vi "performZeroCorrection.vi"(8 "error in (no error)":errorcluster, 9 "Input Range":dbl=10.0 format="%#_10g", 10 "Measurement Function (0: Current)":i32(ring) items=["Current", "Charge", "Voltage", "Resistance"], 11 "Electrometer in":refnum<class "Electrometer.lvclass">) -> (0 "error out":errorcluster, 2 "Set Range":string, 3 "Electrometer out":refnum<class "Electrometer.lvclass">)   [LabVIEW 2016, in "Electrometer.lvclass"]
uses:
  Electrometer.lvclass
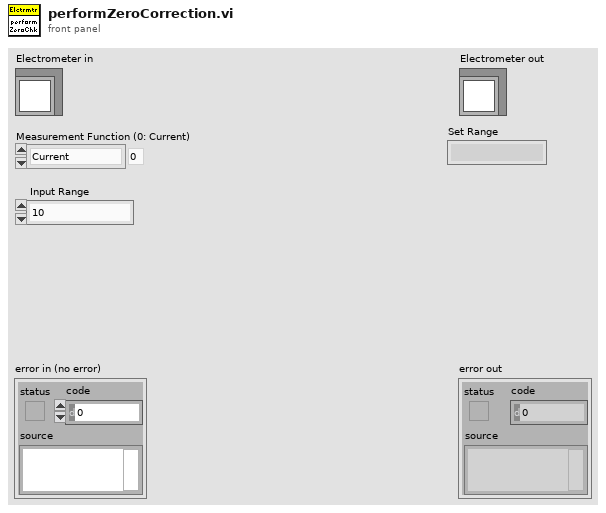
[diagram p1: front panel]
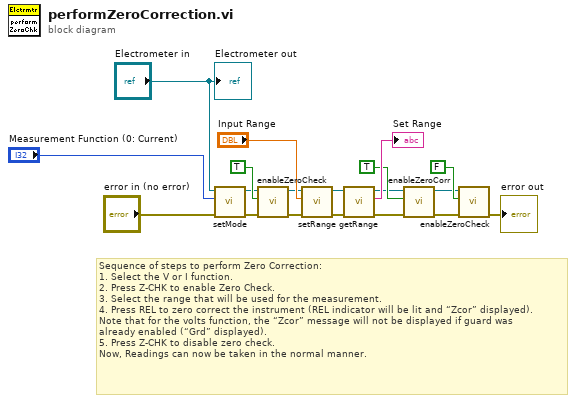
[diagram p0: block diagram]
diagram:
  # "Sequence of steps to perform Zero Correction:\n1. Select the V or I function.\n2. Press Z-CHK to enable Zero Check.\n3. Select the range that will be used for the measurement.\n4. Press REL to zero correct the instrument (REL indicator will be lit and “Zcor” displayed).\nNote that for the volts function, the “Zcor” message will not be displayed if guard was\nalready enabled (“Grd” displayed).\n5. Press Z-CHK to disable zero check.\nNow, Readings can now be taken in the normal manner."
  n1 = call "setMode.vi"("error in (no error)"="error in (no error)", "Measurement Function (0: Current)"="Measurement Function (0: Current)", "Electrometer in"="Electrometer in") -> ("error out"=w15:errorcluster, "Electrometer out"=w17:refnum<class "Electrometer.lvclass">)  [unwired: 7 in]
  n2 = call "enableZeroCheck.vi"("error in (no error)"=w15, "Enable Zero Check (T: Enable)"=TRUE, "Electrometer in"=w17) -> ("error out"=w11:errorcluster, "Electrometer out"=w12:refnum<class "Electrometer.lvclass">)  [unwired: 7 in]
  n3 = call "setRange.vi"("error in (no error)"=w11, "Range"="Input Range", "Electrometer in"=w12) -> ("error out"=w9:errorcluster, "Electrometer out"=w10:refnum<class "Electrometer.lvclass">)  [unwired: 7 in]
  n4 = call "getRange.vi"("error in (no error)"=w9, "Electrometer in"=w10) -> ("error out"=w7:errorcluster, "Range"=→"Set Range":string, "Electrometer out"=w5:refnum<class "Electrometer.lvclass">)  [unwired: 7 in]
  n5 = call "enableZeroCorr.vi"("error in (no error)"=w7, "Enable Zero Correct (T: Enable)"=TRUE, "Electrometer in"=w5) -> ("error out"=w2:errorcluster, "Electrometer out"=w3:refnum<class "Electrometer.lvclass">)  [unwired: 7 in]
  n6 = call "enableZeroCheck.vi"("error in (no error)"=w2, "Enable Zero Check (T: Enable)"=FALSE, "Electrometer in"=w3) -> ("error out"=→"error out":errorcluster)  [unwired: 7 in, 1 out]
  "Electrometer out" <- "Electrometer in"
